vi "Init.vi"(7 "Prepend Result Name":bool, 8 "error in (no error)":errorcluster, 9 "SA Pin":string, 10 "NF Freq (Hz)":string, 11 "Measurement Name":string) -> (0 "error out":errorcluster, 3 "NF out":refnum<class "NF Eval.lvclass">)   [LabVIEW 2016, in "SeqAuto Evaluations.lvlib" / "NF Eval.lvclass"]
uses:
  NF Eval.lvclass
  C:/Sequence Automation/Plugins/SeqAuto IEvaluation.lvlibp/SeqAuto IEvaluation.lvclass
  NF Eval.lvclass/NF Eval.ctl
  Plugins/SeqAuto IEvaluation.lvlibp/Write Measurement Name.vi
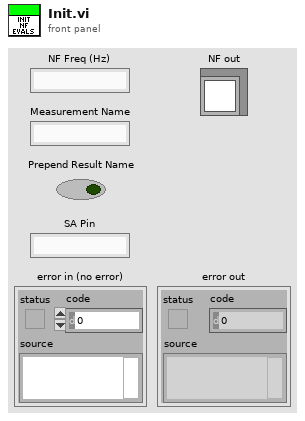
[diagram p1: front panel]
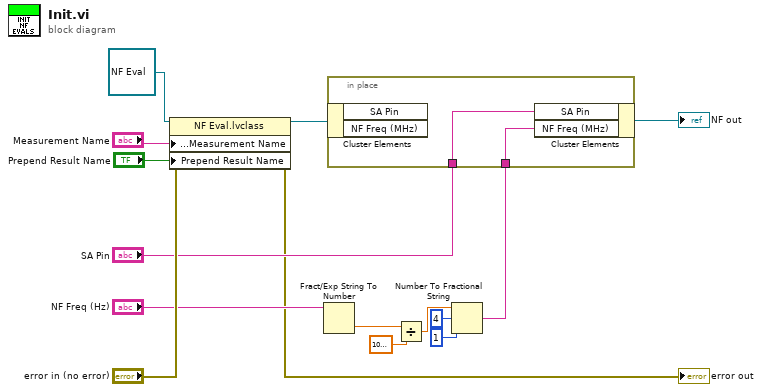
[diagram p0: block diagram]
diagram:
  n1 = property class="NF Eval.lvclass"(reference=refnum<class "NF Eval.lvclass"> refnum ("NF in"), error in="error in (no error)", "Protected Methods:Measurement Name"="Measurement Name", "Prepend Result Name"="Prepend Result Name") -> (reference out=w3:refnum<class "NF Eval.lvclass">, error out=→"error out":errorcluster)
  n2 = Fract/Exp String To Number(string="NF Freq (Hz)") -> (number=w11:dbl)  [unwired: 3 in, 1 out]
  n3 = Divide(x=w11, y=1000000.0) -> (x/y=w9:dbl)
  n4 = Number To Fractional String(number=w9, width (-)=i16 4, precision (6)=i16 1) -> (F-format string=w12:string)  [unwired: 1 in]
  n5 = in-place {
    in-place-border: "SA Pin" -> [w17]
    in-place-border: w12 -> [w16]
    n6 = in-place-cluster #1(w3) -> ()  [unwired: 2 out]
    n7 = in-place-cluster #1("SA Pin"=w17, "NF Freq (MHz)"=w16) -> (→"NF out":refnum<class "NF Eval.lvclass">)
  }
